vi "LS372_Check_Queue.vi"(7 "error in (no error)":errorcluster, 10 "queue":refnum<queue>) -> (0 "error out":errorcluster, 1 "LS372-Control":T1 {"MC Thermometer" items=["Speer 9905", "ROX U02453"]}, 3 "New Entries?":bool)   [LabVIEW 2019]
uses:
  LS372/Ls372-Control.ctl
panel:
  out "Numeric":i32
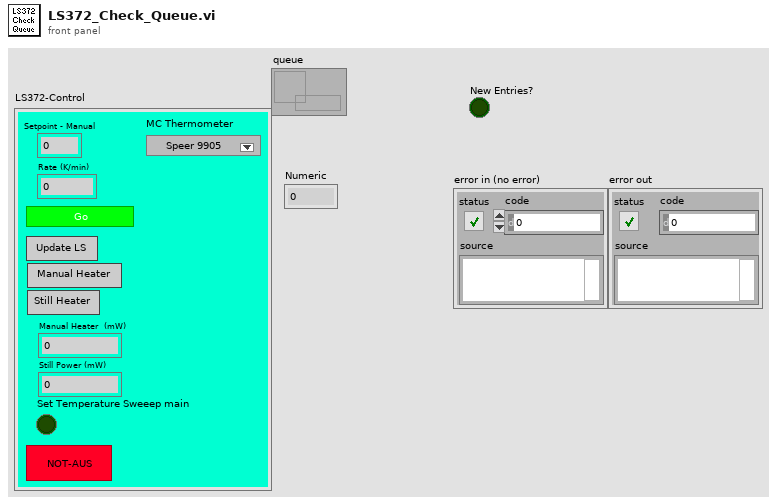
[diagram p1: front panel]
types:
  T1 = typedef "Ls372-Control.ctl" = cluster{"Activate Tsweep":bool, "Setpoint - Manual":dbl, "Rate (K/min)":dbl, "Update Lakeshores":bool, "Still Heater":bool, "Still Power (mW)":dbl, "Manual Heater":bool, "Manual Heater  (mW) ":dbl, "MC Thermometer":u16, "Set Temperature Sweeep main":bool, "Disable Heater":bool}
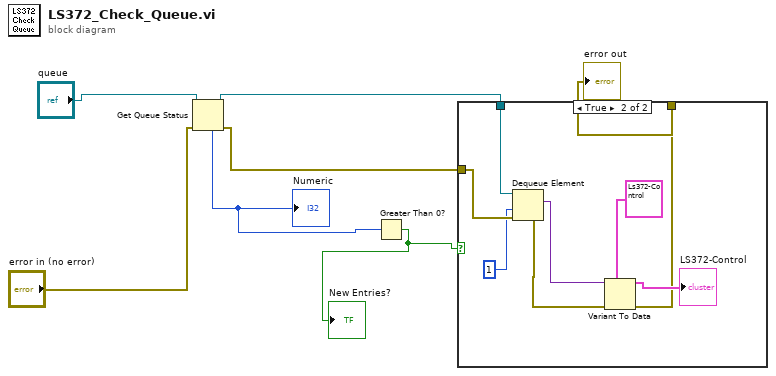
[diagram p0: block diagram]
diagram:
  n1 = Get Queue Status(queue="queue", error in (no error)="error in (no error)") -> (queue out=w6:refnum<queue>, error out=w5:errorcluster, # elements in queue=w3:i32)  [unwired: 1 in, 5 out]
  "Numeric" <- w3
  n2 = Greater Than 0?(x=w3) -> (x > 0?=w2:bool)
  "New Entries?" <- w2
  n3 = case shown="True" w2 {
    tunnel: w6 -> [_ w16]
    tunnel: w5 -> [w8 w15]
    tunnel: [w8 w9] -> w1
    frame False {
    }
    frame True {
      n4 = Dequeue Element(queue=w16, timeout in ms (-1)=1, error in (no error)=w15) -> (element=w13:variant, error out=w12:errorcluster)  [unwired: 2 out]
      n5 = Variant To Data(error in=w12, type=T1 {"Activate Tsweep"=FALSE, "Setpoint - Manual"=0.0, "Rate (K/min)"=0.0, "Update Lakeshores"=FALSE, "Still Heater"=FALSE, "Still Power (mW)"=0.0, "Manual Heater"=FALSE, "Manual Heater  (mW) "=0.0, "MC Thermometer"=0, "Set Temperature Sweeep main"=FALSE, "Disable Heater"=FALSE} ("LS372-Control 2"), Variant=w13) -> (data=→"LS372-Control":T1, error out=w9:errorcluster)
    }
  }
  "error out" <- w1
